vi "AlliGator Logistic Square Gated IRF Characteristics Map.vi"(8 "error in (no error)":errorcluster, 9 "Cursor Names Array":string[](array[string]), 10 "Cursor Positions Array":dbl[](array[numeric]), 11 "AlliGator Internal Variables DVR":refnum<data-value>) -> (0 "error out":errorcluster, 1 "Message":string, 3 "AlliGator Internal Variables DVR":refnum<data-value>)   [LabVIEW 2021, in "AlliGator Scripts.lvlib"]
doc: "Computes the decays of all ROIs and fits them with a logistic square gate model.\n\nSaves the results in an ASCII file."
uses:
  AlliGator Scripts.lvlib
  Globals, Variables, Constants/AlliGator Variables List.ctl
  Globals, Variables, Constants/AlliGator Globals, Variables & Constants.lvlib
  Image/Named ROI Description.ctl
  Image/Image.lvlib
  Decay Analysis/Decay Processing/AlliGator Decay Processing.lvlib
  Source Image/AlliGator Source Image.lvlib
  <vilib>/vision/Image Controls.llb/IMAQ Image.ctl
  <vilib>/ErrorRing/Error Ring.xnode
  Strings/Strings.lvlib
  Time/Time.lvlib
  Decay Analysis/IRF/AlliGator IRF.lvlib
  Fits/Fit Calculation Method.ctl
  Fits/Fits.lvlib
  Fits/Residual Type.ctl
  Fits/Decay Convolution/Decay Model.ctl
  Settings/AlliGator Settings List.ctl
  Settings/AlliGator Settings.lvlib
  Fits/Basic Fit Options.ctl
  Decay Analysis/Decay Preprocessing/AlliGator Decay Preprocessing.lvlib
  GUI/GUI.lvlib
  Globals, Variables, Constants/AlliGator Abort.vi
  Fits/Square Pulse/Square Pulse Levels Type.ctl
  Fits/Square Pulse/Square Pulse Options.ctl
  Fits/Non-linear Fitting Algorithm.ctl
  Utilities/Utilities.lvlib
  Notebook/Notebook.lvlib
  <vilib>/Utility/error.llb/Error Cluster From Error Code.vi
  <vilib>/Utility/file.llb/Write Delimited Spreadsheet (string).vi
  Variant/Variant to Data/Variant to Data.lvlib
  Fits/Non-linear Fitting Method v2.ctl
  Variant/Variant to Data/Variant to U16.vi
  Fits/Optimal Offset Selection Criterion.ctl
  Rich Text Box/Text Format List.ctl
  Fits/IRF(X)PSED/Fit Weights Type v2.ctl
  Fits/IRF(X)PSED/Decay Fit Options v4.ctl
  Phasor/Phasor Reference Series.ctl
  Phasor/Phasor.lvlib
  Phasor/Phasor (g, s).ctl
  Phasor/Calibration Phasor (m, phi).ctl
  Files/AlliGator Data Series Type.ctl
  Files/AlliGator Files.lvlib
  Internal Variables/AlliGator Internal Variables v2.ctl
  Internal Variables/AlliGator Internal Variables.lvlib
  Phasor Graph/AlliGator Decay Metadata v3.ctl
  Phasor Graph/AlliGator Phasor Graph.lvlib
  Phasor Graph/AlliGator Raw Phasor Plot Data v5.ctl
  Decay Analysis/Decay Preprocessing/AlliGator Baseline Subtraction Method.ctl
  Decay Analysis/Decay Preprocessing/AlliGator Decay Background Subtraction Info.ctl
  Graphs/XY Graph/XY Graph Plot Shift Method.ctl
  Graphs/XY Graph/XY Graph Add-Ons.lvlib
  Graphs/XY Graph/XY Graph Plot Shift Parameters.ctl
  Decay Analysis/Decay Preprocessing/AlliGator Decay Extrapolation Parameters.ctl
  Files/AlliGator FLI Dataset Type.ctl
  Phasor/Phasor Harmonic Data.ctl
  Phasor Plot/AlliGator Phasor Multi-Harmonic Data.ctl
  Phasor Plot/AlliGator Phasor Plot.lvlib
  Source Image/AlliGator Displayed Image.ctl
  Fits/IRF(X)PSED/Decay Fit Parameters & Derived Quantities List v2.ctl
  Fits/IRF(X)PSED/Decay Fit Parameters In List.ctl
  Decay Analysis/Decay Fit/AlliGator Decay Fit Parameter Constraints 2.ctl
  Decay Analysis/Decay Fit/AlliGator Decay Fit.lvlib
  Internal Variables/AlliGator Gate Image Set.ctl
  Settings/AlliGator Gate Arithmetic.ctl
  Dual-Channel Datasets/AlliGator Dataset Channel.ctl
  Dual-Channel Datasets/AlliGator Dual-Channel Datasets.lvlib
  Decay Analysis/Decay Preprocessing/AlliGator Decay Preprocessing Parameters.ctl
  Phasor/Phasor Standard Deviation Options.ctl
  Phasor/Phasor Calibration Map v2.ctl
  Fits/IRF(X)PSED/MLE Baseline Offset Type.ctl
  Decay Fit Parameter Map/AlliGator Parameter Maps Data.ctl
  Decay Fit Parameter Map/AlliGator Decay Fit Parameter Map.lvlib
  Fits/IRF(X)PSED/Decay Fit Result Constraint.ctl
  Decay Fit Parameter Map/AlliGator Decay Fit Options & Parameters v4.ctl
panel:
  # "see the AlliGator License on the block diagram (Ctrl+E or Window:Show Block Diagram)"
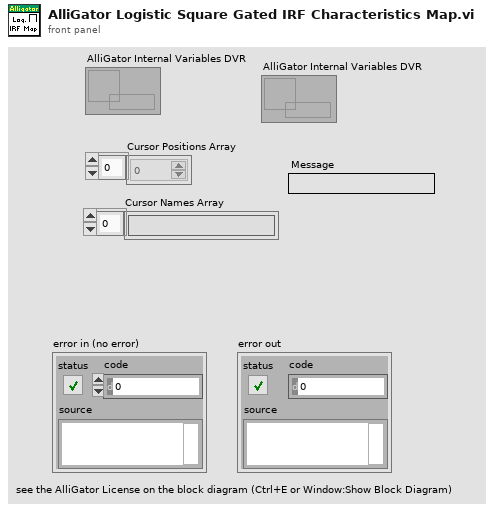
[diagram p1: front panel]
types:
  T1 = typedef "Notebook.lvlib/Text Format List.ctl" = enum16{"Message", "Result", "Error", "Setting", "Verbose", "Warning"}
  T2 = typedef "Fits.lvlib/Optimal Offset Selection Criterion.ctl" = enum16{"Min Chi^2", "Max R^2"}
  T3 = typedef "AlliGator Settings.lvlib/AlliGator Settings List.ctl" = enum16{"GUI:Visible Settings Tab", "GUI:Last Run Version", "Source Image:Use Image Histogram for Contrast", "Source Image:Low Count Pixels Rejection Options", "Source Image:High Count Pixels Rejection Options", "Source Image:Use Image Brightness", "Source Image:Blend Overlay with Image Background", "Source Image:Use Fixed ROI Diameter", "Source Image:ROI Diameter", "Source Image:ROI Center Color", "Source Image:Peak Threshold", "Source Image:Intensity Threshold", "Source Image:Image Binning Options", "Source Image:Image Smoothing Options", "Source Image:Image Histogram Active", "Source Image:Invert Binary Mask", "Source Image:Hot Pixel Removal", "Source Image:Overlay Analyzed ROI Center", "Source Image:Auto-Adjust Contrast", "Source Image:Histogram Lower Percentile", "Source Image:Histogram Upper Percentile", "Source Image:Save Source Image", "Source Image:Scale Bar Options", "Source Image:Image Resolution (Pixel Size)", "Source Image:Flatfield Correction", "Source Image:Show Dead Left Columns Correction", "Source Image:Dead Left Columns Correction", "Source Image:Image Pre-Processing Operations Order", "Source Image:Overlay ROI Median", "Source Image:Median Overlay Color", "Data Information:Gate Width", "Data Information:Nanotime Gate Separation", "Data Information:Macrotime Gate Separation", "Data Information:Gate Step", "Data Information:# Gates", "Data Information:Gate Image Exposure", "Data Information:Gate Image Integration", "Data Information:Gates to Skip", "Data Information:Gates to Keep", "Data Information:Define Gates to", "Data Information:Channel Name", "Data Information:Available Channel Names", "Data Information:Channel Arithmetic", "Data Information:Background File Subtraction", "Data Information:Background File", "Data Information:Background Scaling Factor", "Data Information:Background Pile-up Correction", "Data Information:Background Pixel Well Capacity", "Data Information:Laser Period", "Data Information:SYNC Period", "Data Information:Pile-up Correction", "Data Information:Pixel Well Capacity", "Data Information:Dataset Scaling Factor", "Fluorescence Decay_Decay Pre-Processing:Reverse Gates", "Fluorescence Decay_Decay Pre-Processing:Verbose Decay Pre-Processing", "Fluorescence Decay_Decay Pre-Processing:Use Decay Pre-Processing", "Fluorescence Decay_Decay Pre-Processing:Background Subtraction", "Fluorescence Decay_Decay Pre-Processing:Background Definition Range", "Fluorescence Decay_Decay Pre-Processing:Baseline Subtraction Method", "Fluorescence Decay_Decay Pre-Processing:Decay Pre-Processing Operations Order", "Fluorescence Decay_Decay Pre-Processing:Smoothing Parameter", "Fluorescence Decay_Decay Pre-Processing:Shift Decay", "Fluorescence Decay_Decay Pre-Processing:Decay Shift Parameters", "Fluorescence Decay_Decay Pre-Processing:Fold Decay", "Fluorescence Decay_Decay Pre-Processing:# Folds", "Fluorescence Decay_Decay Pre-Processing:1-Normalize Decay", "Fluorescence Decay_Decay Pre-Processing:[0-1]-Normalize Decay", "Fluorescence Decay_Decay Pre-Processing:Smoothen Decay", "Fluorescence Decay_Decay Pre-Processing:Extrapolate Decay", "Fluorescence Decay_Decay Pre-Processing:Use Periodicity", "Fluorescence Decay_Decay Pre-Processing:Use Cursors", "Fluorescence Decay_Decay Pre-Processing:Tail Fraction", "Fluorescence Decay_Decay Pre-Processing:Head Fraction", "Fluorescence Decay_Decay Pre-Processing:Additional Points", "Fluorescence Decay_Decay Pre-Processing:Straighten Decay", "Fluorescence Decay_Decay Pre-Processing:Constant Background", "Fluorescence Decay_Decay Pre-Processing:Pixel-Normalize Decay", "Fluorescence Decay_Advanced Analysis:Extract IRF instead of Decay", "Fluorescence Decay_Advanced Analysis:IRF Extraction Options", "Fluorescence Decay_Advanced Analysis:IRF Optimization Options", "Fluorescence Decay_Advanced Analysis:Square Pulse Options", "Fluorescence Decay_Advanced Analysis:IRF Order", "Fluorescence Decay_Advanced Analysis:IRF Time Constants", "Fluorescence Decay_Advanced Analysis:Wavelet Analysis Options", "Fluorescence Decay_Advanced Analysis:Average Lifetime Options", "Fluorescence Decay_Fit Options:Fit Options", "Fluorescence Decay_Fit Options:Use Legacy Fitting Approach", "Fluorescence Decay_Fit Options:Use Data Information Laser Period", "Fluorescence Decay_Fit Parameters:Displayed Fit Parameters", "Fluorescence Decay_Fit Parameters:Fit Parameter Constraints", "Fluorescence Decay_Fit Parameters:Export Tabulated Results", "Fluorescence Decay_Fit Parameters:MLE Baseline Offset Type", "Fluorescence Decay_Fit Parameters:MLE Baseline Offset", "Fluorescence Decay_Fit Parameters:Guess Parameter Names", "Fluorescence Decay_Fit Parameters:Guess Parameter Values", "Fluorescence Decay_Fit Parameters:Guess Parameters Options", "Fluorescence Decay_Fit Parameters:Optimal Offset Selection Criterion", "Fluorescence Decay_Styles:Show Last Decay Only", "Fluorescence Decay_Styles:Decay Graph Color Array", "Fluorescence Decay:Decay Graph Active", "Fluorescence Decay Statistics:Min Peak Value", "Fluorescence Decay Statistics:Reject Low Decay Peak Pixels", "Fluorescence Decay Statistics:Reject High Decay Peak Pixels", "Fluorescence Decay Statistics:Max Peak Value", "Time Traces:Use File Timestamp", "Time Traces:Time Step", "Time Traces:Use Intensity Correction File", "Time Traces:Intensity Correction File", "Phasor Plot:Phasor Plot Smoothing Options", "Phasor Plot:Phasor Plot Size", "Phasor Plot:Phasor Plot Graphics Options", "Phasor Plot:Cumulative Phasor Plot", "Phasor Plot:Use Phasor Brightness", "Phasor Plot:Blend Overlay with Phasor Background", "Phasor Plot:Save Phasor Plot", "Phasor Plot:Show References", "Phasor Plot:Phasor Ratio Decay Range", "Phasor Plot:Exponential Fading", "Phasor Plot:Phasor Ratio Reference Colors", "Phasor Plot:Reference Radius", "Phasor Plot:Show Color Map Vertices", "Phasor Plot:Phasor Plot Active", "Phasor Plot:Phasor Ratio Color Map Type", "Phasor Plot:Phasor Ratio Color Map", "Phasor Plot:Phasor Ratio Display Range", "Phasor Plot:Selected Image ROI(s)", "Phasor Plot:All Image ROIs", "Phasor Plot:Selected Phasor Plot ROI(s)", "Phasor Plot:All Phasor Plot ROIs", "Phasor Plot:Phasor Ratio Color-Coded Quantity", "Phasor Plot:Store Phasor Harmonics", "Phasor Plot:Draw Reference Segment", "Phasor Plot:User-Defined Quantity", "Phasor Plot:Color Scale High Color", "Phasor Plot:Color Scale Low Color", "Phasor Plot:Intensity-weighted Phasor Plot", "Phasor Graph:Phasor Frequency", "Phasor Graph:Phasor Ratio Type", "Phasor Graph:Pixel-level Phasor Computation", "Phasor Graph:Save Phasor Graph", "Phasor Graph:Phasor Graph Active", "Phasor Graph:Phasor SDV Options", "Phasor Graph:Intensity-weighted Phasor Graph", "Phasor Graph:Define Shortest Lifetime as", "Phasor Calibration:Use Backup Calibration if needed", "Phasor Calibration:Backup Calibration Type", "Phasor Calibration:Calibration Type", "Phasor Calibration:Calibration Lifetime", "Phasor Calibration:Calibration Map Algorithm", "Single-Exponential Phasor Locus (SEPL):Gate Parameters", "Single-Exponential Phasor Locus (SEPL):User-defined Gate", "Single-Exponential Phasor Locus (SEPL):User-defined IRF", "Single-Exponential Phasor Locus (SEPL):Phasor Parameters", "Single-Exponential Phasor Locus (SEPL):Decay & IRF Parameters", "Single-Exponential Phasor Locus (SEPL):Display Parameters", "Lifetime Analysis:Decay Analysis Parameters", "Lifetime Analysis:Lifetime Map Active", "Plugins:Python Settings", "Miscellaneous:Verbose Mode", "Miscellaneous:Beep after Script", "Miscellaneous:Saved Image File Format", "Miscellaneous:Exported Gate Image Settings", "Miscellaneous:Include Loading in Timing", "Miscellaneous:Verbose Settings Mode", "Miscellaneous:Histogram Options", "Miscellaneous:Beep on Error", "Miscellaneous:# Logical Processors Used", "Miscellaneous:ROI Description Max Characters", "Miscellaneous:Verbose Error Mode", "Miscellaneous:Transparent Mask Color"}
  T4 = typedef "AlliGator Globals, Variables & Constants.lvlib/AlliGator Variables List.ctl" = enum16{"---- GUI ----", "GUI:Initialization Status", "GUI:State Indicators Refnum", "GUI:Original AlliGator Menu Items", "GUI:Current Action Loop State", "GUI:Script in progress", "GUI:Playback", "GUI:Loop Playback", "GUI:Search ROI Used", "GUI:Search ROI", "Decay Graph Max Legend Size", "Intensity Graph Max Legend Size", "Decay Statistics Graph Max Legend Size", "Phasor Graph Max Legend Size", "Phasor Ratio Graph Max Legend Size", "Lifetime Graph Max Legend Size", "---- Files ----", "Files:Export Dataset Frames as Individual Files", "Files:Show Batch Export Help Balloons", "Files:Frames in Dataset", "Files:ptu File Frame Start Indices", "Files:Current Frame in Dataset", "Files:Current Frame Timestamp", "Files:Dataset Loaded", "Files:Dataset Metadata", "Files:Dataset Channel", "Files:Dataset Data Description", "Files:Background Dataset Metadata", "Files:Background Dataset Channel", "Files:Background Dataset Data Description", "Files:Background File Subtraction", "Files:Background File Path", "Files:Background File Pile-up Correction", "Files:Background File Pixel Well Capacity", "Files:Background File Scaling Factor", "Files:Current Dataset Load Settings", "Files:Dataset Path", "Files:ICCD-specific Information", "Files:Macrotime Gate Separation", "------ Python Plugins ------", "Python Plugins:Information", "Python Plugins:Python Session", "Python Plugins:Valid Python Session?", "---- Source Image ----", "Source Image:ROIs", "Source Image:Current ROI", "Source Image:ROI Event Refnum", "X_Source Image:Display Range", "X_Source Image:Palette Information", "X_Source Image:Type of Displayed Image", "X_Time Gate Slider", "Source Image:Palette List", "Source Image:Scale", "Source Image:ROI Overlay Color", "Source Image:Overlay to Erase", "Source Image:Is Displayed Image Accumulated", "Source Image:White Light Image Modified", "Source Image:Mask Image Modified", "---- Image Profile Window ----", "Image Profile:Window Event Refnum", "Image Profile:IntensityType", "Image Profile:Intensity Average Type", "Image Profile:Intensity-weighted SDV", "Image Profile:Box Profile Type", "Image Profile:Window Open", "Image Profile:Plotted Fit Parameter", "------ Phasor Graph -------", "Phasor Graph:Show Line", "---- Phasor Plot ---", "Phasor Plot:Parameters Changed", "Phasor Plot:FLI Dataset Modified since last Calculation", "Phasor Harmonics Data", "Selected Phasor Harmonics", "Phasor Harmonic Manager Event Refnum", "Phasor Plot:ROIs", "Phasor Plot:Current ROI", "Phasor Plot:ROI Event Refnum", "Phasor Plot:Image Reference Points", "Phasor Plot:Computed", "Phasor Plot:Palette Information", "Phasor Plot:Palette List", "Phasor Plot:Phasor Ratio Palette Information", "Phasor Plot:Phasor Ratio Palette List", "Phasor Plot:Image Scale", "Phasor Plot:Image Overlay to Erase", "Phasor Plot:Image Elements to Update", "Phasor Plot:Current Calculation Parameters", "Phasor Plot:Current Calibration Options", "Phasor Plot:Reset Cumulated Phasor Plot", "Phasor Plot:Reference 1", "Phasor Plot:Lifetime Reference 1", "Phasor Plot:Reference 1 Frequency", "Phasor Plot:Reference 2", "Phasor Plot:Lifetime Reference 2", "Phasor Plot:Reference 2 Frequency", "---- Decay Analysis ----", "Number of Selected Decays to Fit", "LS Fit Results", "LAR Fit Results", "BS Fit Results", "Last Decay Max - Min", "Best Fit Parameters", "Best Fit Parameter Names", "Actual Size X", "Actual Size Y", "Binning X", "Binning Y", "Actual # Gates", "Dataset Number", "Gates to...", "Gates Skipped", "Gates to keep", "Gate Step", "Gate Separation", "Reversed Gates", "Pile-up Correction", "Pixel Well Capacity", "Background Subtracted", "Background Subtraction Method", "Background Definition Range", "Background File (deprecated)", "Number of Dataset Accumulated", "Array of Accumulated Dataset Paths", "Do Averaged Datasets", "Destination File Path", "Process Plot Target", "Use 1/D as Phasor Frequency", "---- Decay Fit Parameter Map -----", "Decay Fit Parameter Map:Palette Information", "Decay Fit Parameter Map:Palette List", "Decay Fit Parameter Map:X Resolution", "Decay Fit Parameter Map:Y Resolution", "Decay Fit Parameter Map:Use Decay Fit Result Constraints", "Decay Fit Parameter Map:Decay Fit Result Constraints", "Decay Fit Parameter Map:Decay Fit Result Constraints Applied", "---- Parameter Map ----", "Parameter Map:Palette Information", "Parameter Map:Palette List", "------- Local Decay Window ---------", "Local Decay Graph Window:Event Refnum", "Local Decay Graph Window:Use normalized IRF for convolution", "----- Miscellaneous ----", "Misc:Skippable Dialog Windows Status"}
  T5 = typedef "IMAQ Image.ctl" = refnum<image>
  T6 = typedef "Fits.lvlib/Square Pulse Options.ctl" = cluster{"Method":T7, "# Bins":i32, "Threshold %":dbl, "Center on Midpoint":bool, "Smoothen Plot":bool}
  T7 = typedef "Fits.lvlib/Square Pulse Levels Type.ctl" = enum16{"Mode", "Mean"}
  T8 = typedef "Fits.lvlib/Basic Fit Options.ctl" = cluster{"Fitting Method":T9, "Weighted Fit":T10, "Residual Type":T11, "Compute Parameter Uncertainties":bool, "Fitting Algorithm":T12}
  T9 = typedef "Fits.lvlib/Non-linear Fitting Method v2.ctl" = enum16{"Least Square", "Least Absolute Residual", "Bisquare", "MLE", "-", "Best of All"}
  T10 = typedef "Fits.lvlib/Fit Weights Type v2.ctl" = enum16{"Unweighted", "1/Variance (Neyman)", "1/Variance (Pearson)", "Best of All"}
  T11 = typedef "Fits.lvlib/Residual Type.ctl" = enum16{"Standard", "Normalized", "Reduced"}
  T12 = typedef "Fits.lvlib/Non-linear Fitting Algorithm.ctl" = enum16{"Levenberg-Marquardt", "Trust-Region Dogleg"}
  T13 = typedef "Fits.lvlib/Decay Fit Options v4.ctl" = cluster{"Show Fit Residuals":bool, "Fit Model":T14, "Residual Type":T11, "Max Decay Percentile":dbl, "Min Decay Percentile":dbl, "Show Full Decay":bool, "Weights":T10, "Fitting Method":T9, "Compute Parameter Uncertainties":bool, "Periodic Boundaries":bool, "Model Calculation":T15, "Period":dbl[unit], "Termination Criteria":cluster{"Max Iterations":i32, "Max Function Calls":i32, "Max Time":dbl[unit], "Function Tolerance":dbl, "Parameter Tolerance":dbl, "Gradient Tolerance":dbl, "Min Lambda":dbl, "Max Lambda":dbl, "Initial Tick Count":u32}, "Offset Resolution":dbl[unit], "Use Local IRF":bool, "Fitting Algorithm":T12, "Show Confidence Interval ":bool, "Confidence Level":dbl}
  T14 = typedef "Fits.lvlib/Decay Model.ctl" = enum16{"1-Exponential", "2-Exponentials"}
  T15 = typedef "Fits.lvlib/Fit Calculation Method.ctl" = enum16{"Simulation", "Convolution", "Integration"}
  T16 = typedef "Image.lvlib/Named ROI Description.ctl" = cluster{"ROI Descriptor":T17, "ROI Name":string, "Overlay Color":u32}
  T17 = typedef "ROI Descriptor" = cluster{"Global Rectangle":i32[], "Contours":cluster{"ID":enum32{"External", "Internal"}, "Type":u32, "Coordinates":i32[]}[]}
  T18 = typedef "AlliGator Internal Variables.lvlib/AlliGator Internal Variables v2.ctl" = cluster{"----------------------------- Images -----------------------------":u8, "Displayed Image":T5, "White Light Image":T5, "Mask Image":T5, "ROI Mask Image":T5, "Current Dataset Images 1":T19, "Background Dataset Images 1":T19, "Current Dataset Images 2":T19, "Background Dataset Images 2":T19, "Current Dataset Arithmetic Images":T19, "Accumulated Dataset Images 1":T19, "Accumulated Dataset Images 2":T19, "Accumulated Dataset Arithmetic Images":T19, "----------------------------- File Paths -----------------------------":u8, "Phasor Plot Image":T5, "Decay Fit Parameter Map Image":T5, "Parameter Map Image":T5, "Single Data Point Path":path, "White Light Image Path":path, "Mask Image Path":path, "Time-Series Folder":path, "[Time-Series Paths]":path[], "----------------------------- FLI Dataset -----------------------------":u8, "Current Dataset":i32, "Single Dataset Type":T20, "Current Folder":string, "AlliGator Data Series Type":T21, "# Datasets":i32, "Dual-Channel Dataset":bool, "Selected Channel Name":string, "Dataset Channel":T22, "Channel Arithmetic":T23, "Dual-Channel Background Dataset":bool, "Background Channel":T22, "Dual-Channel Accumulated Dataset":bool, "Start Time":dbl, "[Time-Series Timestamps]":dbl[], "[Intensity Corrections]":dbl[], "Time Series Script":bool, "Type of Displayed Image":T24, "Gate Image Slide":u16, "# Gates":i32, "ROIs":T16[], "----------------------------- Decays -----------------------------":u8, "ROI Decay":cluster{"t Array":dbl[], "I Array":dbl[]}, "Valid Decay":bool, "Decay  Metadata":T25, "Reference Decay Plot Name":string, "Reference Decay":cluster{"t Array":dbl[], "I Array":dbl[]}, "Decay Shift Plot":cluster{"Time Stamps":dbl[], "Decay Shifts":dbl[]}, "[Decays Max Values]":sgl[], "[Decays Min Values]":sgl[], "----------------------------- Calibration -----------------------------":u8, "Calibration Phasor":T31, "Calibration Phasor Series":T32, "Phasor Calibration Map":T33, "Calibration Map MD5 Digest":string, "----------------------------- Phasor Graph -----------------------------":u8, "Last Raw Phasor":T34, "Last Calibrated Phasor":T34, "Last Calibrated Phasor SDV":T34, "Phasor Graph:Phasor Plot":cluster{"g Array":dbl[], "s Array":dbl[]}, "Phasor Graph:Phasor SDV Plot":cluster{"g Array":dbl[], "s Array":dbl[]}, "[Phasor Graph:Raw Phasor Plots]":T35[], "Phasor Plot locked to Ref 1":i32, "[Phasor Plot(s) locked to Ref 1]":i32[], "[Phasor Plot(s) locked to Ref 2]":i32[], "[Pixel Phasors]":T34[], "----------------------------- Phasor Plot -----------------------------":u8, "[[Sum Image]]":dbl[][], "[[CSG Phasors]]":csg[][], "[[Valid Pixel?]]":bool[][], "[[Phasor Ratios]]":dbl[][], "[[Average Lifetimes]]":dbl[][], "Amplitude Weighted Average Lifetime":bool, "I/m/phi Dataset":cluster{"I/m/phi Dataset?":bool, "Base Frequency":dbl[unit], "Harmonic Orders":u8[]}, "Multi Phasor Plot Data":T37, "----------------------------- Decay Fit Parameter Map -----------------------------":u8, "Decay Fit Options & Parameters":T39, "Fit Options: Decay Preprocessing Parameters":T43, "Fit Options: Reference Decay":cluster{"t Array":dbl[], "I Array":dbl[]}, "Is Full Image Parameters Map":bool, "Is Single-Pixels Parameters Map":bool, "NLSF Parameters Map X Resolution":i32, "NLSF Parameters Map Y Resolution":i32, "[Single Decay Fit Parameters]":dbl[], "Fit Model":T14, "[[Multiple Decays Fit Parameters]]":dbl[][], "[[Multiple Decays Fit Parameter SDVs]]":dbl[][], "[[IRFs]]":dbl[][], "[ROI Descriptors]":T17[], "IRF Array Time Axis":dbl[], "Decay Array Time Axis":dbl[], "[Decay Fit Parameter Names]":T44[], "[Decay Sum]":dbl[], "Array of Decay Fit Result Constraints":T45[], "Selected ROIs Array":bool[], "----------------------------- Parameter Maps -----------------------------":u8, "[Map Set Names]":string[], "[Parameter Maps]":T46[], "[[User-defined Quantities]]":dbl[][], "User-defined Quantity":string}
  T19 = typedef "AlliGator Internal Variables.lvlib/AlliGator Gate Image Set.ctl" = cluster{"SGL Image Max":T5, "SGL Image Sum":T5, "SGL Gate Images":T5[], "SGL Image Min":T5}
  T20 = typedef "AlliGator Files.lvlib/AlliGator FLI Dataset Type.ctl" = enum16{"HDF5 FLI Dataset", "Gate Image Folder", ".sdt FLI Dataset (Becker & Hickl)", ".ptu FLI Dataset (PicoQuant)", "SS1 FLI Dataset", "SS2 FLI Dataset", "I/m/phi Dataset", ".bin FLI Dataset (PicoQuant Binned)", ".bin FLI Dataset (Piccolo Binned)", ".mat FLI Dataset"}
  T21 = typedef "AlliGator Files.lvlib/AlliGator Data Series Type.ctl" = enum16{"Not a Supported Series", "Gate Images Folder Series", "SwissSPAD 2 Dataset Series", "B&H FLI Dataset Series", "PicoQuant PTU FLI Dataset Series", "PicoQuant BIN FLI Dataset Series", "Piccolo hist BIN FLI Dataset Series", "HDF5 FLI Dataset Series"}
  T22 = typedef "AlliGator Dual-Channel Datasets.lvlib/AlliGator Dataset Channel.ctl" = enum16{"G2", "INT"}
  T23 = typedef "AlliGator Settings.lvlib/AlliGator Gate Arithmetic.ctl" = enum16{"None", "INT-G2", "G2/INT*<INT>", "(1 - G2/INT)*<INT>"}
  T24 = typedef "AlliGator Source Image.lvlib/AlliGator Displayed Image.ctl" = enum16{"Single Gate", "Sum of All Gates", "Max of All Gates", "Min of All Gates", "-", "White Ligth Image", "Mask Image"}
  T25 = typedef "AlliGator Phasor Graph.lvlib/AlliGator Decay Metadata v3.ctl" = cluster{"ROI Descriptor":T17, "ROI Center":cluster{"X":i32, "Y":i32}, "Decay Background Subtraction Info":T26, "Decay Reverted":bool, "Decay Smoothened":bool, "Decay Straightened":bool, "Fitted Tau (Decay Straightening)":dbl, "Decay Shift Parameters":T28, "Decay Shifted":bool, "Decay Extrapolated":bool, "Decay Extrapolation Parameters":T30, "Decay Normalized":bool, "Fold Decay":bool, "# Folds":u32}
  T26 = typedef "AlliGator Decay Preprocessing.lvlib/AlliGator Decay Background Subtraction Info.ctl" = cluster{"Laser Period":dbl[unit], "Gate Duration":dbl[unit], "Baseline Subtraction Method":T27, "Background Definition Range":cluster{"Min Gate":dbl[unit], "Max Gate":dbl[unit]}, "Total Intensity w/o Bkgd Subtraction":dbl, "Bkgd-subtracted Intensity (exp)":dbl, "# Data Points":i32, "Background/Gate":dbl, "Fitted Lifetime":dbl[unit], "Bkgd-subtracted Intensity (theo)":dbl}
  T27 = typedef "AlliGator Decay Preprocessing.lvlib/AlliGator Baseline Subtraction Method.ctl" = enum16{"Mean", "Min", "Square Gated Single-Exponential", "File", "Constant"}
  T28 = typedef "XY Graph Add-Ons.lvlib/XY Graph Plot Shift Parameters.ctl" = cluster{"Type":T29, "Shift":dbl[unit], "Threshold":dbl, "Rotate":bool}
  T29 = typedef "XY Graph Add-Ons.lvlib/XY Graph Plot Shift Method.ctl" = enum16{"Default", "CFD", "Threshold", "Cross-Correlation"}
  T30 = typedef "AlliGator Decay Preprocessing.lvlib/AlliGator Decay Extrapolation Parameters.ctl" = cluster{"Additional Points":u32, "Head Fraction":dbl, "Fitted Tau":dbl, "Use Periodicity":bool, "Use Cursors":bool, "Tail Fraction":dbl}
  T31 = typedef "Phasor.lvlib/Calibration Phasor (m, phi).ctl" = cluster{"m":dbl, "phi":dbl, "Phasor Frequency":dbl[unit], "Reference Lifetime":dbl[unit]}
  T32 = typedef "Phasor.lvlib/Phasor Reference Series.ctl" = cluster{"m Array":dbl[], "phi Array":dbl[], "Phasor Frequency":dbl[unit], "Calibration Lifetime":dbl[unit]}
  T33 = typedef "Phasor.lvlib/Phasor Calibration Map v2.ctl" = cluster{"Phasor Frequency":dbl[unit], "Calibration Lifetime":dbl[unit], "ROI Centers":cluster{"X":i32, "Y":i32}[], "ROI Descriptors":T17[], "Map Resolution X":i32, "Map Resolution Y":i32, "z Array":cdb[]}
  T34 = typedef "Phasor.lvlib/Phasor (g, s).ctl" = cluster{"g":dbl, "s":dbl}
  T35 = typedef "AlliGator Phasor Graph.lvlib/AlliGator Raw Phasor Plot Data v5.ctl" = cluster{"Phasor Plot Name":string, "Raw Phasor Plot":T34[], "Phasor Frequency":dbl[unit], "[Decay Metadata]":T25[], "Raw Phasor Plot SDV":T34[], "Phasor SDV Options":T36, "[Calibration Phasor]":T31[], "Intensity Array":dbl[]}
  T36 = typedef "Phasor.lvlib/Phasor Standard Deviation Options.ctl" = cluster{"Compute Estimated SDV":bool, "# Replicas":u32, "Use Estimated Average Phasor":bool}
  T37 = typedef "AlliGator Phasor Plot.lvlib/AlliGator Phasor Multi-Harmonic Data.ctl" = cluster{"Base Frequency":dbl[unit], "# Harmonics":u8, "Harmonic Orders":u8[], "Phasor Plot Settings Checksum":u64, "Phasor Harmonic Data Array":T38[]}
  T38 = typedef "Phasor.lvlib/Phasor Harmonic Data.ctl" = cluster{"Phasor Harmonic Name":string, "Phasor Plot Settings Checksum":u64, "Phasor Frequency":dbl[unit], "Base Frequency":dbl[unit], "Harmonic Order":u8, "Phasor Plot Parameters":string, "Phasor Array [[CSG]]":csg[][], "Dataset File Path":path}
  T39 = typedef "AlliGator Decay Fit Parameter Map.lvlib/AlliGator Decay Fit Options & Parameters v4.ctl" = cluster{"SYNC Period":dbl[unit], "Fit Options":T13, "Fit Parameter Constraints":T40[], "MLE Baseline Offset":dbl, "MLE Baseline Offset Type":T42}
  T40 = typedef "AlliGator Decay Fit.lvlib/AlliGator Decay Fit Parameter Constraints 2.ctl" = cluster{"Fit Parameter":T41, "Min Value":dbl, "Max Value":dbl, "Global":bool, "Used":bool}
  T41 = typedef "Fits.lvlib/Decay Fit Parameters In List.ctl" = enum16{"Offset", "Baseline", "A_1", "tau_1", "A_2", "tau_2"}
  T42 = typedef "Fits.lvlib/MLE Baseline Offset Type.ctl" = enum32{"Absolute", "Percentage"}
  T43 = typedef "AlliGator Decay Preprocessing.lvlib/AlliGator Decay Preprocessing Parameters.ctl" = cluster{"Background Subtraction":bool, "Straighten Decay":bool, "Reverse Gates":bool, "1-Normalized Decay":bool, "Smoothen Decay":bool, "Smoothing Parameter":dbl, "Shift Decay":bool, "Decay Shift Parameters":T28, "Extrapolate Decay":bool, "Additional Points":u32, "Head Fraction":dbl, "Pixel-Normalize Decay":bool, "Use Periodicity":bool, "Use Cursors":bool, "Tail Fraction":dbl, "Use Decay Pre-Processing":bool, "Fold Decay":bool, "# Folds":u32, "[0-1]-Normalized Decay":bool}
  T44 = typedef "Fits.lvlib/Decay Fit Parameters & Derived Quantities List v2.ctl" = enum16{"Offset", "Baseline", "A_1", "tau_1", "A_2", "tau_2", "<tau>_a", "f1_a", "f2_a", "<tau>_i", "f1_i", "f2_i", "-", "R^2", "Chi^2"}
  T45 = typedef "Fits.lvlib/Decay Fit Result Constraint.ctl" = cluster{"Fit Parameter":enum16{"Offset", "Baseline", "A_1", "tau_1", "A_2", "tau_2", "<tau>_a", "f1_a", "f2_a", "<tau>_i", "f1_i", "f2_i", "-", "R^2", "Chi^2", "Max Relative Residual", "<Residual ACF>", "Residual ACF SDV", "tau_2/tau_1"}, "Min Value":dbl, "Max Value":dbl, "Use Constraint":bool}
  T46 = typedef "AlliGator Decay Fit Parameter Map.lvlib/AlliGator Parameter Maps Data.ctl" = cluster{"Map Set Name":string, "[Parameter Names]":string[], "[[Parameters]]":dbl[][], "[[Parameter SDVs]]":dbl[][], "Decay Array Time Axis":dbl[], "[[IRFs]]":dbl[][], "IRF Array Time Axis":dbl[], "X Resolution":i32, "Y Resolution":i32, "Intensity Array":dbl[]}
  T47 = typedef "AlliGator Settings.lvlib/AlliGator Pixel Counts Constraints.ctl" = cluster{"High Count Pixels Rejection Options":T48, "Low Count Pixels Rejection Options":T49}
  T48 = typedef "AlliGator Settings.lvlib/AlliGator High Count Pixels Rejection Options.ctl" = cluster{"Background High Threshold Factor":dbl, "Fixed High Background Threshold":dbl, "Reject High Count Pixels":bool, "High Percentile":dbl}
  T49 = typedef "AlliGator Settings.lvlib/AlliGator Low Count Pixels Rejection Options.ctl" = cluster{"Background Low Threshold Factor":dbl, "Fixed Low Background Threshold":dbl, "Reject Low Count Pixels":bool, "Low Percentile":dbl}
  T50 = cluster{"Decay Peak Constraint":bool, "Min":dbl, "Max":dbl}
  T51 = typedef "Rich Text Box.lvlib/Text Formatting.ctl" = cluster{"Font":string, "Text Color":T52, "Background Color":T52, "Style":T53, "Font Size":dbl, "Alignment":T54}
  T52 = typedef "Rich Text Box.lvlib/Text Colors.ctl" = enum16{"Unchanged", "Black", "Blue", "Cyan", "Maroon", "Gray", "Violet", "Green", "Light Green", "Orange", "Yellow", "Magenta", "Red", "White"}
  T53 = typedef "Rich Text Box.lvlib/Text Style.ctl" = enum16{"Regular", "Bold", "Italic", "Underline", "Strikeout"}
  T54 = typedef "Rich Text Box.lvlib/Text Alignment.ctl" = enum16{"Left", "Right", "Center"}
  T55 = cluster{"t Axis":dbl[], "ROI Intensity Array":dbl[]}
  T56 = typedef "Fits.lvlib/Non-linear Fit Output v4.ctl" = cluster{"best nonlinear fit":dbl[], "best fit parameters":dbl[], "R^2":dbl, "RMSE":dbl, "error out":errorcluster, "Fitting Method":T57, "number of function calls":i32, "number of iterations":i32, "covariance":T58, "Chi 2":dbl, "DOF":i32, "Fit Convergence Criterion":T59, "Fitting Algorithm":T12, "Weighted Fit":T10, "Gradient":dbl, "|Delta Chi 2|":dbl, "|Delta Chi 2|/Chi 2":dbl, "Max |Delta a| /|a|":dbl, "Lambda":dbl, "RSS":dbl, "AIC":dbl, "BIC":dbl, "Max number of function calls":i32, "Max number of iterations":i32, "IRF":T60, "IRF Normalization Factor":dbl, "Decay Normalization Factor":dbl, "Number of offset fits":i32, "Weighted Chi2":dbl, "Unweighted Chi2":dbl}
  T57 = typedef "Fits.lvlib/Nonlinear Fit Method.ctl" = enum16{"Least Square", "Least Absolute Residual", "Bisquare", "MLE"}
  T58 = typedef "NI_Matrix.lvlib/RealMatrix.ctl" = dbl[][]
  T59 = typedef "Fits.lvlib/Convergence Criteria.ctl" = enum16{"Continue", "Tolerances Exceeded", "Max Time Exceeded", "Max Iterations Exceeded", "Max Function Evaluations Exceeded", "Scale Range Exceeded"}
  T60 = typedef "XY Graph Add-Ons.lvlib/XY Graph Plot Data.ctl" = cluster{"X Array":dbl[], "Y Array":dbl[]}
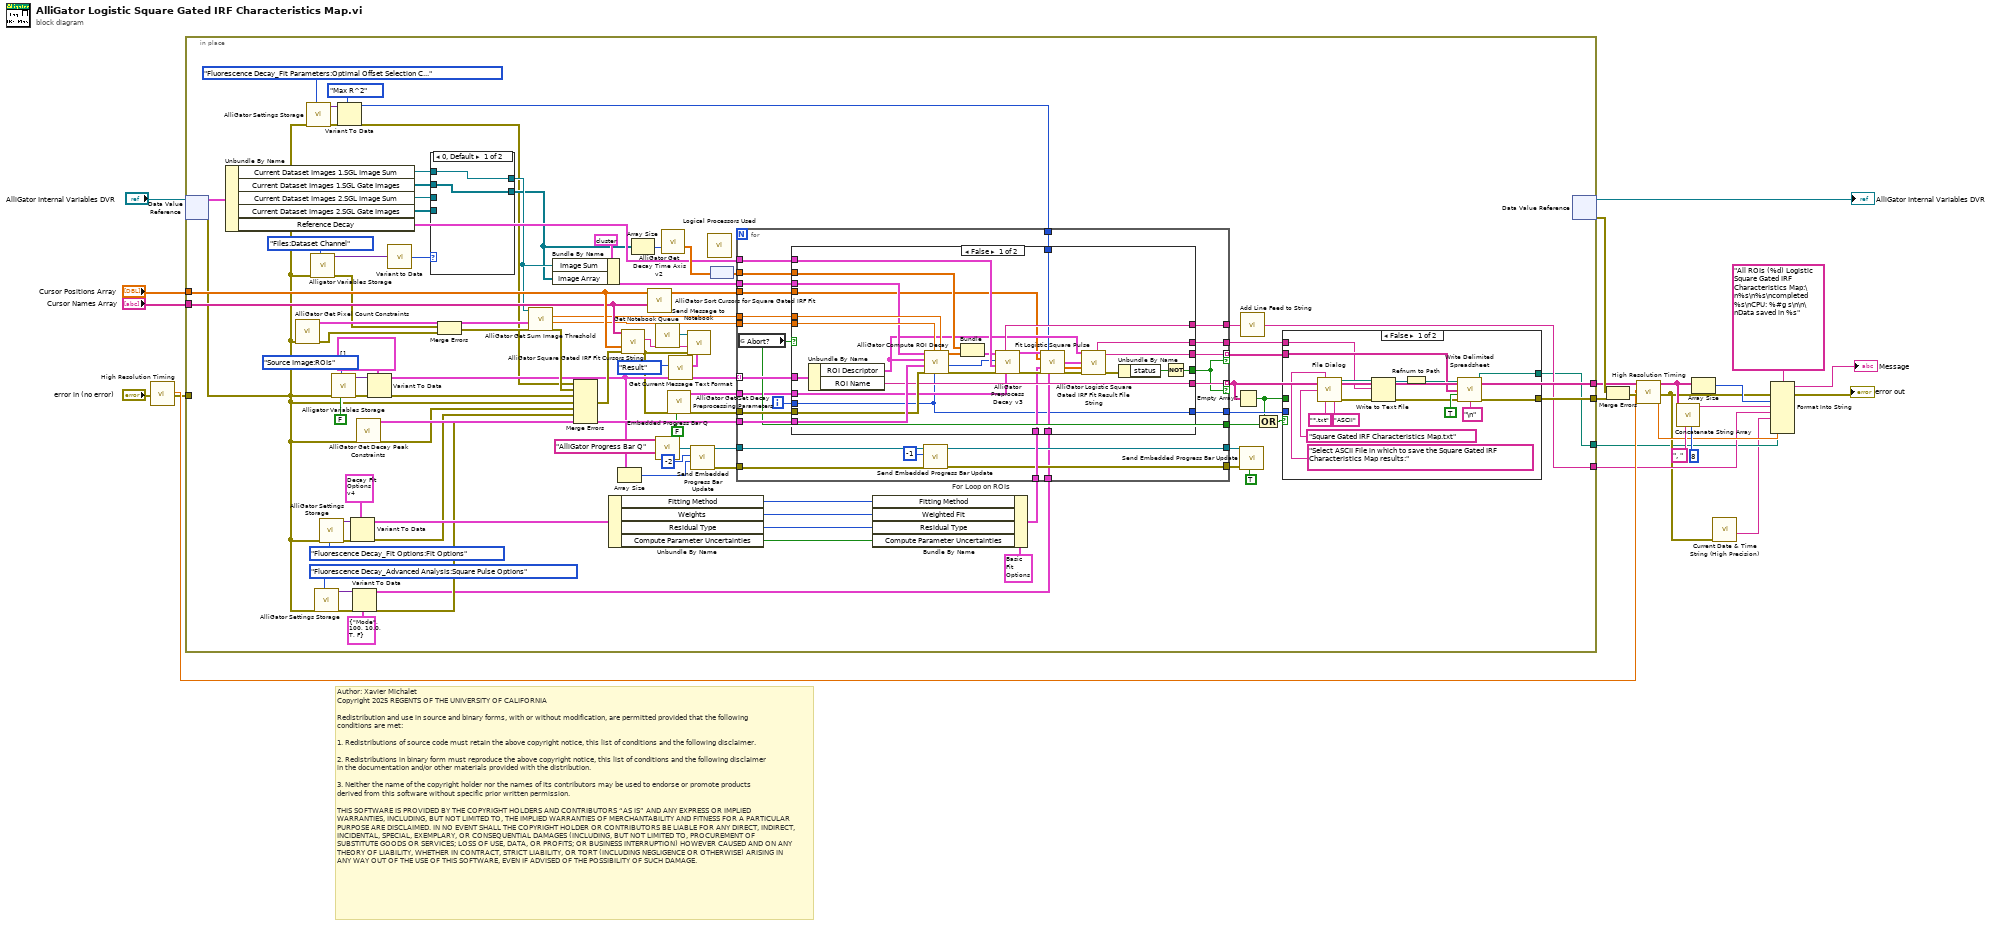
[diagram p0: block diagram]
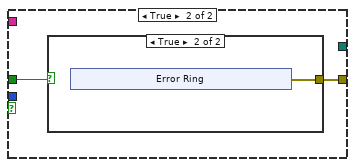
[diagram p3: hidden frame]
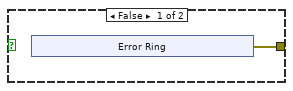
[diagram p4: hidden frame]
diagram:
  # "Author: Xavier Michalet\nCopyright 2025 REGENTS OF THE UNIVERSITY OF CALIFORNIA\n\nRedistribution and use in source and binary forms, with or without modification, are permitted provided that the following conditions are met:\n\n1. Redistributions of source code must retain the above copyright notice, this list of conditions and the following disclaimer.\n\n2. Redistributions in binary form must reproduce the above copyright notice, this list of conditions and the following disclaimer in the documentation and/or other materials provided with the distribution.\n\n3. Neither the name of the copyright holder nor the names of its contributors may be used to endorse or promote products derived from this software without specific prior written permission.\n\nTHIS SOFTWARE IS PROVIDED BY THE COPYRIGHT HOLDERS AND CONTRIBUTORS “AS IS” AND ANY EXPRESS OR IMPLIED WARRANTIES, INCLUDING, BUT NOT LIMITED TO, THE IMPLIED WARRANTIES OF MERCHANTABILITY AND FITNESS FOR A PARTICULAR PURPOSE ARE DISCLAIMED. IN NO EVENT SHALL THE COPYRIGHT HOLDER OR CONTRIBUTORS BE LIABLE FOR ANY DIRECT, INDIRECT, INCIDENTAL, SPECIAL, EXEMPLARY, OR CONSEQUENTIAL DAMAGES (INCLUDING, BUT NOT LIMITED TO, PROCUREMENT OF SUBSTITUTE GOODS OR SERVICES; LOSS OF USE, DATA, OR PROFITS; OR BUSINESS INTERRUPTION) HOWEVER CAUSED AND ON ANY THEORY OF LIABILITY, WHETHER IN CONTRACT, STRICT LIABILITY, OR TORT (INCLUDING NEGLIGENCE OR OTHERWISE) ARISING IN ANY WAY OUT OF THE USE OF THIS SOFTWARE, EVEN IF ADVISED OF THE POSSIBILITY OF SUCH DAMAGE."
  n1 = call "High Resolution Timing.vi"("Error In"="error in (no error)") -> ("elapsed (relative) seconds"=w14:dbl, "Error Out"=w9:errorcluster)  [unwired: 16 in, 1 out]
  n2 = in-place {
    in-place-border: [w110] -> w19
    in-place-border: [w109] -> w11
    in-place-border: w9 -> [_]
    in-place-border: [w108] -> w8
    in-place-border: "Cursor Positions Array" -> [w107]
    in-place-border: "Cursor Names Array" -> [w106]
    in-place-border: [w105] -> w4
    n3 = in-place-dvr #1("AlliGator Internal Variables DVR") -> (w111:T18, w29:errorcluster)
    n4 = Unbundle By Name(w111) -> ("Current Dataset Images 1.SGL Image Sum"=w47:T5, "Current Dataset Images 1.SGL Gate Images"=w48:T5[], "Current Dataset Images 2.SGL Image Sum"=w43:T5, "Current Dataset Images 2.SGL Gate Images"=w44:T5[], "Reference Decay"=w90:cluster{"t Array":dbl[], "I Array":dbl[]})
    n5 = call "AlliGator Get Pixel Count Constraints.vi"("error in (no error)"=w29) -> ("error out"=w98:errorcluster, "Pixel Count Constraints"=w99:T47)  [unwired: 9 in]
    n6 = call "AlliGator Settings Storage.vi"("AlliGator Settings List"=AlliGator_Settings_List."Fluorescence Decay_Fit Parameters:Optimal Offset Selection Criterion", "Error In"=w29) -> ("Error Out"=w31:errorcluster, "Variant Data out"=w32:variant)  [unwired: 8 in]
    n7 = call "Alligator Variables Storage.vi"("AlliGator Variable"=AlliGator_Variables_List."Files:Dataset Channel" ("Alligator Variable"), "Error In"=w29) -> ("Error Out"=w34:errorcluster, "Data out"=w36:variant)  [unwired: 7 in, 1 out]
    n8 = call "AlliGator Settings Storage.vi"("AlliGator Settings List"=AlliGator_Settings_List."Fluorescence Decay_Advanced Analysis:Square Pulse Options", "Error In"=w29) -> ("Error Out"=w56:errorcluster, "Variant Data out"=w57:variant)  [unwired: 8 in]
    n9 = call "AlliGator Settings Storage.vi"("AlliGator Settings List"=AlliGator_Settings_List."Fluorescence Decay_Fit Options:Fit Options", "Error In"=w29) -> ("Error Out"=w73:errorcluster, "Variant Data out"=w71:variant)  [unwired: 8 in]
    n10 = call "Alligator Variables Storage.vi"("Get(F)/Set"=FALSE, "AlliGator Variable"=AlliGator_Variables_List."Source Image:ROIs" ("Alligator Variable"), "Error In"=w29) -> ("Error Out"=w102:errorcluster, "Data out"=w103:variant)  [unwired: 6 in, 1 out]
    n11 = Variant To Data(error in=w31, type=Optimal_Offset_Selection_Criterion."Max R^2" ("Optimal Offset Selection Criterion"), Variant=w32) -> (data=w27:T2, error out=w26:errorcluster)
    n12 = Variant To Data(error in=w73, type=T13 {"Show Fit Residuals"=TRUE, "Fit Model"=enum."1-Exponential", "Residual Type"=enum."Standard", "Max Decay Percentile"=0.0, "Min Decay Percentile"=0.0, "Show Full Decay"=TRUE, "Weights"=enum."Unweighted", "Fitting Method"=enum."Least Square", "Compute Parameter Uncertainties"=TRUE, "Periodic Boundaries"=TRUE, "Model Calculation"=enum."Simulation", "Period"=1.2500000000000001e-08, "Termination Criteria"={"Max Iterations"=1000, "Max Function Calls"=0, "Max Time"=1000.0, "Function Tolerance"=1e-06, "Parameter Tolerance"=1e-06, "Gradient Tolerance"=0.0, "Min Lambda"=1e-06, "Max Lambda"=1e-06, "Initial Tick Count"=0}, "Offset Resolution"=1.2500000000000001e-08, "Use Local IRF"=TRUE, "Fitting Algorithm"=enum."Levenberg-Marquardt", "Show Confidence Interval "=TRUE, "Confidence Level"=95.0} ("Fit Options"), Variant=w71) -> (data=w74:T13, error out=w70:errorcluster)
    n13 = Variant To Data(error in=w56, type=T6 {"Method"=enum."Mode", "# Bins"=100, "Threshold %"=10.0, "Center on Midpoint"=TRUE, "Smoothen Plot"=FALSE} ("Square Pulse Options"), Variant=w57) -> (data=w52:T6, error out=w53:errorcluster)
    n14 = call "AlliGator Get Decay Peak Constraints.vi"("error in (no error)"=w29) -> ("Error Out"=w83:errorcluster, "Decay Peak Constraints"=w94:T50)  [unwired: 9 in]
    n15 = Variant To Data(error in=w102, type=T16[] [] ("Stored ROIs in"), Variant=w103) -> (data=w60:T16[], error out=w97:errorcluster)
    n16 = call-poly "Variant to Data.vi"("Variant"=w36) -> ("U16 Value"=w33:u16)  [unwired: 8 in]
    n17 = case shown="0, Default" w33 {
      tunnel: [w113 w115] -> w45
      tunnel: w44 -> [_ w115]
      tunnel: [w112 w114] -> w46
      tunnel: w43 -> [_ w114]
      tunnel: w48 -> [w113 _]
      tunnel: w47 -> [w112 _]
      frame 0, Default {
      }
      frame 1 {
      }
    }
    n18 = Merge Errors(w34, w98) -> (w35:errorcluster)
    n19 = call "AlliGator Get Sum Image Threshold.vi"("error in (no error)"=w35, "Pixel Counts Constraints"=w99, "Image in"=w46) -> ("error out"=w85:errorcluster, "Pixel Threshold Low"=w95:sgl, "Pixel Threshold High"=w96:sgl)  [unwired: 2 in, 4 out]
    n20 = Bundle By Name(cluster=cluster{"Image Sum":T5, "Image Array":T5[]} {"Image Sum"=refnum, "Image Array"=[]} ("Images"), "Image Sum"=w46, "Image Array"=w45) -> (w93:cluster{"Image Sum":T5, "Image Array":T5[]})
    n21 = Merge Errors(w26, w85, w97, w29, w83, w70, w53) -> (w80:errorcluster)
    n22 = Unbundle By Name(w74) -> ("Fitting Method"=w75:T9, "Weights"=w24:T10, "Residual Type"=w76:T11, "Compute Parameter Uncertainties"=w77:bool)
    n23 = Array Size(array=w60) -> (size(s)=w59:i32)
    n24 = call "AlliGator Square Gated IRF Fit Cursors String.vi"("Error In"=w80, "Cursor Positions Array"=w107, "Cursor Names Array"=w106) -> ("Error Out"=w40:errorcluster, "Message"=w39:string)  [unwired: 7 in]
    n25 = Array Size(array=w45) -> (size(s)=w92:i32)
    n26 = call "AlliGator Sort Cursors for Square Gated IRF Fit.vi"("Cursor Name Array in"=w106, "Cursor Position Array in"=w107) -> ()  [unwired: 8 in, 2 out]
    n27 = call "Get Notebook Queue.vi"() -> ("Notebook Queue"=w41:refnum<queue>)  [unwired: 9 in]
    n28 = call "Embedded Progress Bar Q.vi"("Progress Bar Queue Name"="AlliGator Progress Bar Q") -> ("Progress Bar Queue"=w66:refnum<queue>)  [unwired: 6 in]
    n29 = call "AlliGator Get Decay Time Axis v2.vi"("Number of Gates"=w92) -> ("t Array"=w91:dbl[unit][])  [unwired: 14 in]
    n30 = call "AlliGator Get-Set Decay Preprocessing Parameters.vi"("Get (F)/Set"=FALSE, "Error In"=w40) -> ("Error Out"=w68:errorcluster, "Decay Preprocessing Parameters out"=w50:T43)  [unwired: 8 in]
    n31 = call "Get Current Message Text Format.vi"("Text Format"=Text_Format_List."Result") -> ("Message Formatting"=w42:T51)  [unwired: 8 in, 1 out]
    n32 = call "Send Message to Notebook.vi"("Text Formatting"=w42, "Error In"=w40, "Text"=w39, "Notebook Queue"=w41) -> ()  [unwired: 4 in, 2 out]
    n33 = call "Send Embedded Progress Bar Update.vi"("Max Iterations N"=w59, "Current Iteration i (i or -1: standard or || iteration; 0 or -2: first standard or || iteration)"=-2 ("Current Iteration i (i or -1: standard or || iteration; 0 or -2: first standard or || iteration)"), "Progress Bar Queue in"=w66) -> ("Error Out"=w64:errorcluster, "Progress Bar Queue out"=w65:refnum<queue>)  [unwired: 7 in]
    n34 = call "Logical Processors Used.vi"() -> ()  [unwired: 6 in, 1 out]
    n35 = node(w91) -> (w84:dbl[])
    n36 = Bundle By Name(cluster=T8 {"Fitting Method"=enum."Least Square", "Weighted Fit"=enum."Unweighted", "Residual Type"=enum."Standard", "Compute Parameter Uncertainties"=FALSE, "Fitting Algorithm"=enum."Levenberg-Marquardt"} ("Basic Fit Options"), "Fitting Method"=w75, "Weighted Fit"=w24, "Residual Type"=w76, "Compute Parameter Uncertainties"=w77) -> (w69:T8)
    n37 = for "For Loop on ROIs" {
      tunnel: w60 -> [w168] mode=indexing
      tunnel: w96 -> [w167]
      tunnel: w95 -> [w166]
      tunnel: w93 -> [w165]
      tunnel: w94 -> [w164]
      tunnel: [w148] -> w89
      tunnel: w84 -> [w160]
      tunnel: w90 -> [w161]
      tunnel: [w144] -> w88
      tunnel: [w162] -> w109 mode=indexing if=w157
      tunnel: w68 -> [w163]
      tunnel: [w159] -> w86
      tunnel: w107 -> [w155]
      tunnel: [w158] -> w82 mode=indexing if=w157
      tunnel: [w156] -> w81
      tunnel: w69 -> [w154]
      tunnel: w65 -> [w153]
      tunnel: w64 -> [w152]
      tunnel: [w151] -> w63
      tunnel: [w150] -> w62
      tunnel: w52 -> [w147]
      tunnel: w50 -> [w146]
      tunnel: w27 -> [w143]
      i -> [w145]
      n38 = global read "AlliGator Abort.vi" "Abort?"() -> (w148:bool)
      n39 = case shown="False" w148 {
        tunnel: w168 -> [w199 _]
        tunnel: w167 -> [w198 _]
        tunnel: w166 -> [w197 _]
        tunnel: w165 -> [w196 _]
        tunnel: w164 -> [w195 _]
        tunnel: w163 -> [w194 _]
        tunnel: [w193 _] -> w162
        tunnel: w161 -> [w191 _]
        tunnel: w160 -> [w189 _]
        tunnel: [w186 _] -> w159
        tunnel: [w180 _] -> w158
        tunnel: [w179 _] -> w157
        tunnel: [w177 _] -> w156
        tunnel: w155 -> [w176 _]
        tunnel: w154 -> [w175 _]
        tunnel: w147 -> [w172 _]
        tunnel: w146 -> [w171 _]
        tunnel: w145 -> [w170 _]
        tunnel: [w170 _] -> w144
        tunnel: w143 -> [w169 _]
        frame False {
          n40 = Unbundle By Name(w199) -> ("ROI Descriptor"=w178:T17, "ROI Name"=w193:string)
          n41 = call "AlliGator Compute ROI Decay.vi"("Pixel Threshold High"=w198, "Loop ID"=w170, "Pixel Threshold Low"=w197, "error in (no error)"=w194, "Decay Peak  Constraints"=w195, "ROI Descriptor"=w178, "Images"=w196) -> ("error out"=w190:errorcluster, "# Valid Pixels"=w173:i32, "Decay Points"=w188:dbl[])  [unwired: 2 out]
          n42 = Bundle(w189, "Decay Points"=w188) -> (w187:cluster{dbl[], "Decay Points":dbl[]})  [unwired: 1 in]
          n43 = call "AlliGator Preprocess Decay v3.vi"("Decay Preprocessing Parameters"=w171, "Error In"=w190, "Time-Gated Reference Decay"=w191, "# Pixels"=w173, "Decay (in)"=w187) -> ("Error Out"=w185:errorcluster, "Decay (out)"=w184:T55, "Message"=w186:string)  [unwired: 3 in, 1 out]
          n44 = call "Fit Logistic Square Pulse.vi"("Decay"=w184, "Optimal Offset Selection Criterion"=w169, "Boundaries"=w176, "Basic Fit Options"=w175, "error in (no error)"=w185, "Square Pulse Options"=w172) -> ("Fit Output"=w174:T56, "Delta Best Fit Parameters"=w181:dbl[], "error out"=w183:errorcluster)  [unwired: 5 in, 2 out]
          n45 = call "AlliGator Logistic Square Gated IRF Fit Result File String.vi"("error in (no error)"=w183, "Delta Best Fit Parameters"=w181, "Fit Output"=w174, "ROI Descriptor"=w178) -> ("error out"=w182:errorcluster, "Result String"=w180:string, "Header String"=w177:string)  [unwired: 5 in]
          n46 = Unbundle By Name(w182) -> ("status"=w192:bool)
          n47 = Not(x=w192) -> (.not. x?=w179:bool)
        }
        frame True {
        }
      }
      n48 = call "Send Embedded Progress Bar Update.vi"("Error In"=w152, "Current Iteration i (i or -1: standard or || iteration; 0 or -2: first standard or || iteration)"=-1 ("Current Iteration i (i or -1: standard or || iteration; 0 or -2: first standard or || iteration)"), "Progress Bar Queue in"=w153) -> ("Error Out"=w150:errorcluster, "Progress Bar Queue out"=w151:refnum<queue>)  [unwired: 7 in]
    }
    n49 = Empty Array?(array=w109) -> (empty?=w38:bool)
    n50 = call "Send Embedded Progress Bar Update.vi"("Stop Progress Bar (F)"=TRUE ("Hide Progress Bar (F)"), "Error In"=w62, "Progress Bar Queue in"=w63) -> ()  [unwired: 7 in, 2 out]
    n51 = call "Add Line Feed to String.vi"("String"=w86) -> ("String\\n"=w108:string)  [unwired: 8 in]
    n52 = Compound Arithmetic op=OR(w38, w89) -> (w87:bool)
    n53 = case shown="False" w87 {
      tunnel: [w120 w132] -> w110
      tunnel: w88 -> [_ _]
      tunnel: w82 -> [w123 _]
      tunnel: w81 -> [w117 _]
      tunnel: [w116 _] -> w105
      tunnel: w38 -> [_ w131]
      frame False {
        n54 = call "File Dialog"("prompt"="Select ASCII File in which to save the Square Gated IRF Characteristics Map results:" ("prompt (Choose or enter file path)"), "default name"="Square Gated IRF Characteristics Map.txt", "pattern (all files)"="*.txt", "pattern label"="ASCII") -> ("selected path"=w125:path, "error out"=w130:errorcluster)  [unwired: 8 in, 2 out]
        n55 = Write to Text File(file (use dialog)=w125, text=w117, error in=w130) -> (refnum out=w119:refnum<file>, error out=w121:errorcluster)  [unwired: 1 in, 1 out]
        n56 = Refnum to Path(1:w119) -> (0:w118:path)
        n57 = call-poly <vilib>:"Write Delimited Spreadsheet.vi"("file path (dialog if empty)"=w118, "1D data"=w123, "append to file? (new file:F)"=TRUE, "error in (no error)"=w121, "delimiter (\\t)"="\n" ("delimiter (\\t)")) -> ("new file path (Not A Path if cancelled)"=w116:path, "error out"=w120:errorcluster)  [unwired: 9 in]
      }
      frame True {
        n58 = case shown="True" w131 {
          tunnel: [w133 w138] -> w132
          frame False {
            n59 = xnode "Error Ring"() -> ("error out"=w133:errorcluster)
          }
          frame True {
            n60 = xnode "Error Ring"() -> ("error out"=w138:errorcluster)
          }
        }
      }
    }
    n61 = in-place-dvr #1() -> (→"AlliGator Internal Variables DVR":refnum<data-value>, w20:errorcluster)  [unwired: 1 in]
  }
  n62 = Merge Errors(w20, w19) -> (w16:errorcluster)
  n63 = call "High Resolution Timing.vi"("relative seconds (NaN)"=w14, "Error In"=w16) -> ("elapsed (relative) seconds"=w13:dbl, "Error Out"=w7:errorcluster)  [unwired: 15 in, 1 out]
  n64 = call "Concatenate String Array.vi"("Max Number of Elements (None: -1)"=8 ("Max Number of Elements (None: 1)"), "Separator (TAB)"=", ", "String Array"=w11) -> ("Formatted String"=w12:string)  [unwired: 8 in]
  n65 = Array Size(array=w11) -> (size(s)=w10:i32)
  n66 = call "Current Date & Time String (High Precision).vi"("Error In"=w7) -> ("on <Date> at <Time>"=w1:string)  [unwired: 7 in, 3 out]
  n67 = Format Into String(format string="All ROIs (%d) Logistic Square Gated IRF Characteristics Map:\n%s\n%s\ncompleted %s\nCPU: %#g s\n\n\nData saved in %s", error in=w7, w10, w12, w8, w1, w13, w4) -> (resulting string=→"Message":string, error out=→"error out":errorcluster)  [unwired: 1 in]
